vi "Mag calib routine.vi"(7 "Norm field":sgl format="%#_13g", 8 "Error In":errorcluster, 10 "Uncalibrated data":sgl[][](array[numeric])) -> (0 "Error Out":errorcluster, 1 "Calib data":T1, 2 "Calib data":sgl[](array[numeric]), 3 "Ainverse":sgl[][](array[numeric]))   [LabVIEW 2016]
uses:
  Typedef/Mag bit depth.ctl
  <vilib>/Analysis/Matrix/Datatypes/RealMatrix.ctl
  <vilib>/Analysis/baseanly.llb/Real A x B.vi
  <vilib>/Analysis/_algsub.llb/Real PseudoInverse Matrix.vi
  <vilib>/Analysis/7linalg.llb/Real Matrix Square Root.vi
  <vilib>/Analysis/7linalg.llb/Real Transpose Matrix.vi
  <vilib>/Analysis/Matrix/Numeric/Conversions/Array To Matrix - RA2.vi
  <vilib>/Analysis/Matrix/Numeric/Subtract/Subtract - RM,RM.vi
  <vilib>/Analysis/baseanly.llb/Real Inverse Matrix.vi
  <vilib>/Analysis/7linalg.llb/Real Eigenvalues and Vectors.vi
  <vilib>/Analysis/Matrix/Numeric/Absolute Value/Absolute Value - CM.vi
  <vilib>/Analysis/Matrix/Numeric/Subtract/Subtract (Elementwise) - RM,R.vi
  <vilib>/Analysis/Matrix/Numeric/Square Root/Square Root - RM.vi
  <vilib>/Analysis/Matrix/Numeric/Conversions/Matrix To Array - RM.vi
  <vilib>/Analysis/Matrix/Numeric/Multiply/Multiply - CM,C.vi
  <vilib>/Analysis/Matrix/Numeric/Conversions/Matrix To Array - CM.vi
  <vilib>/Analysis/Matrix/NI_Matrix.lvlib
  <vilib>/Analysis/NI_AALBase.lvlib
  <vilib>/Analysis/NI_AALPro.lvlib
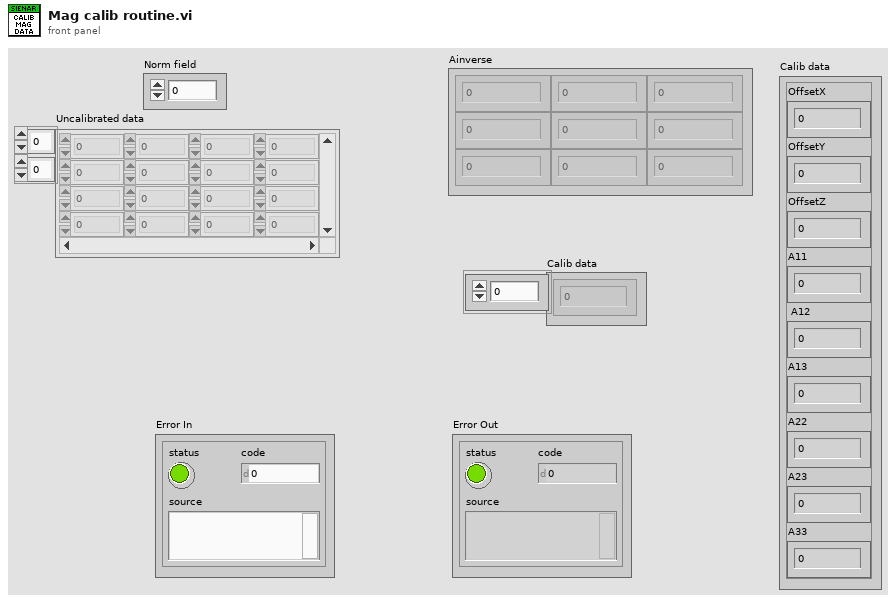
[diagram p1: front panel]
types:
  T1 = cluster{"OffsetX":i16, "OffsetY":i16, "OffsetZ":i16, "A11":sgl, " A12":sgl, "A13":sgl, "A22":sgl, "A23":sgl, "A33":sgl}
  T2 = typedef "Mag bit depth.ctl" = enum16{"14bit", "16bit"}
  T3 = typedef "NI_Matrix.lvlib/RealMatrix.ctl" = dbl[][]
  T4 = typedef "NI_Matrix.lvlib/ComplexMatrix.ctl" = cdb[][]
  T5 = cluster{i16, i16, i16, "Complex Matrix Element":sgl, "Complex Matrix Element":sgl, "Complex Matrix Element":sgl, "Complex Matrix Element":sgl, "Complex Matrix Element":sgl, "Complex Matrix Element":sgl}
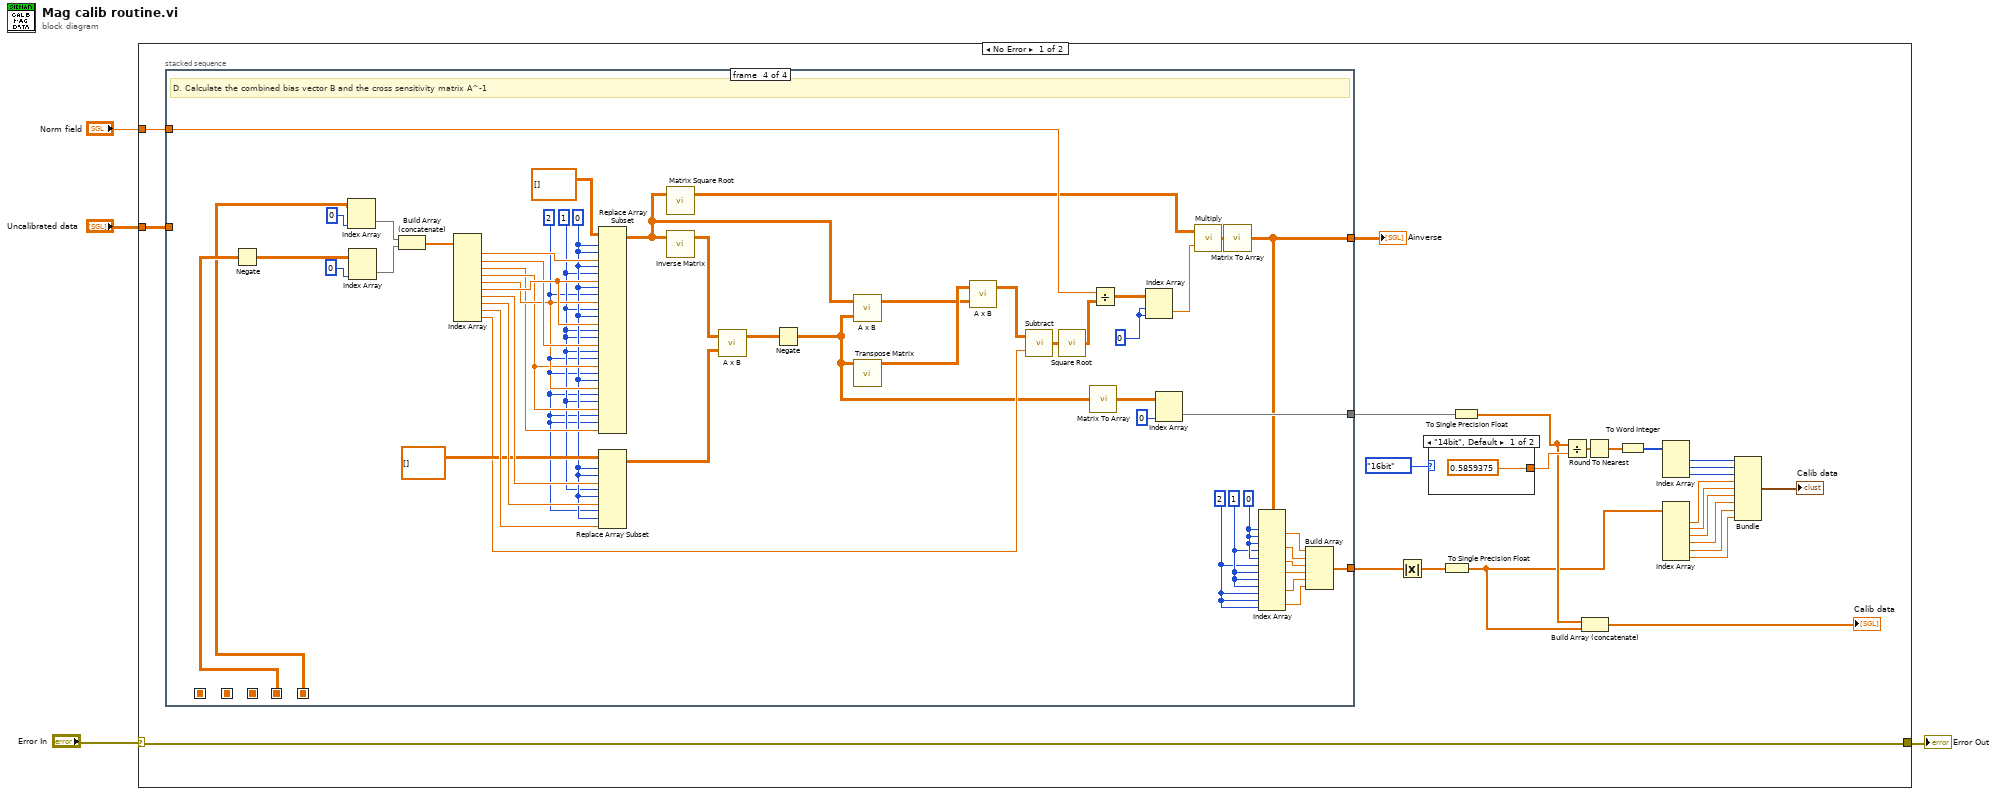
[diagram p0: block diagram]
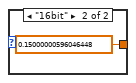
[diagram p2: hidden frame]
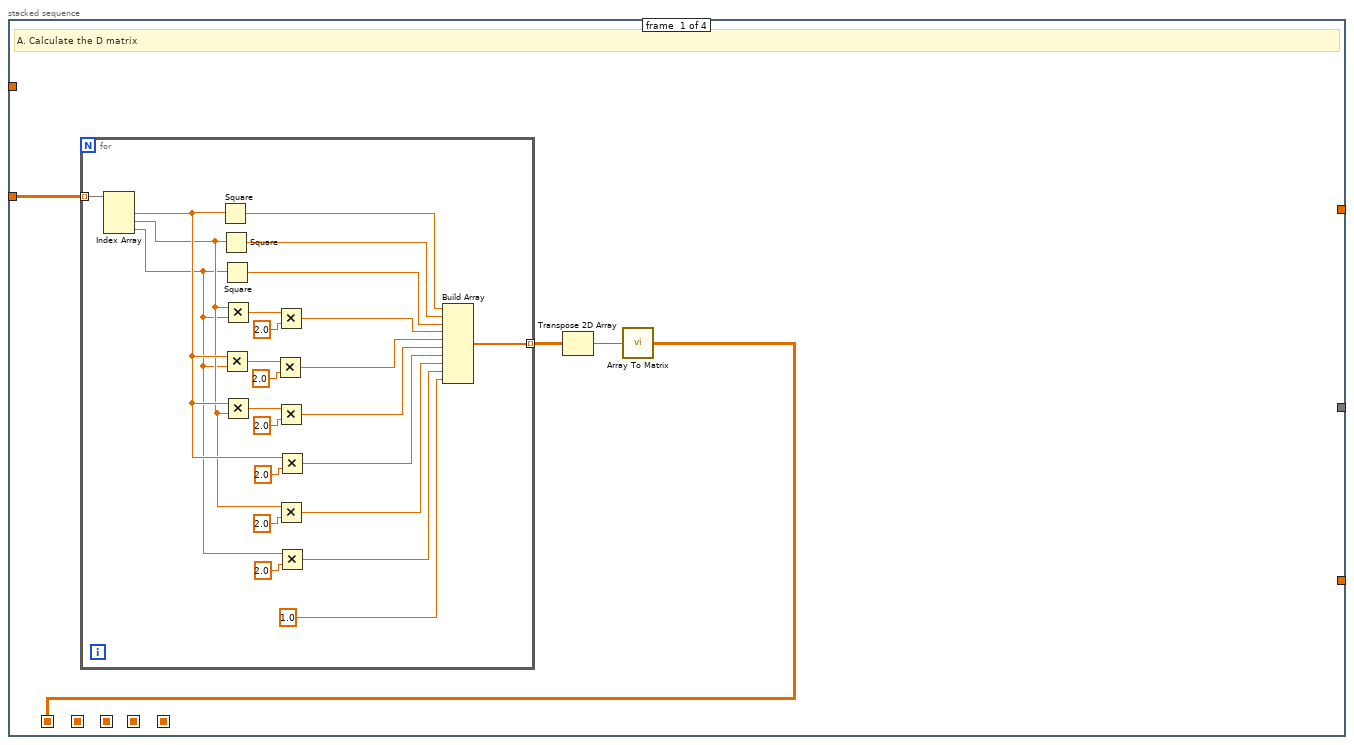
[diagram p3: hidden frame]
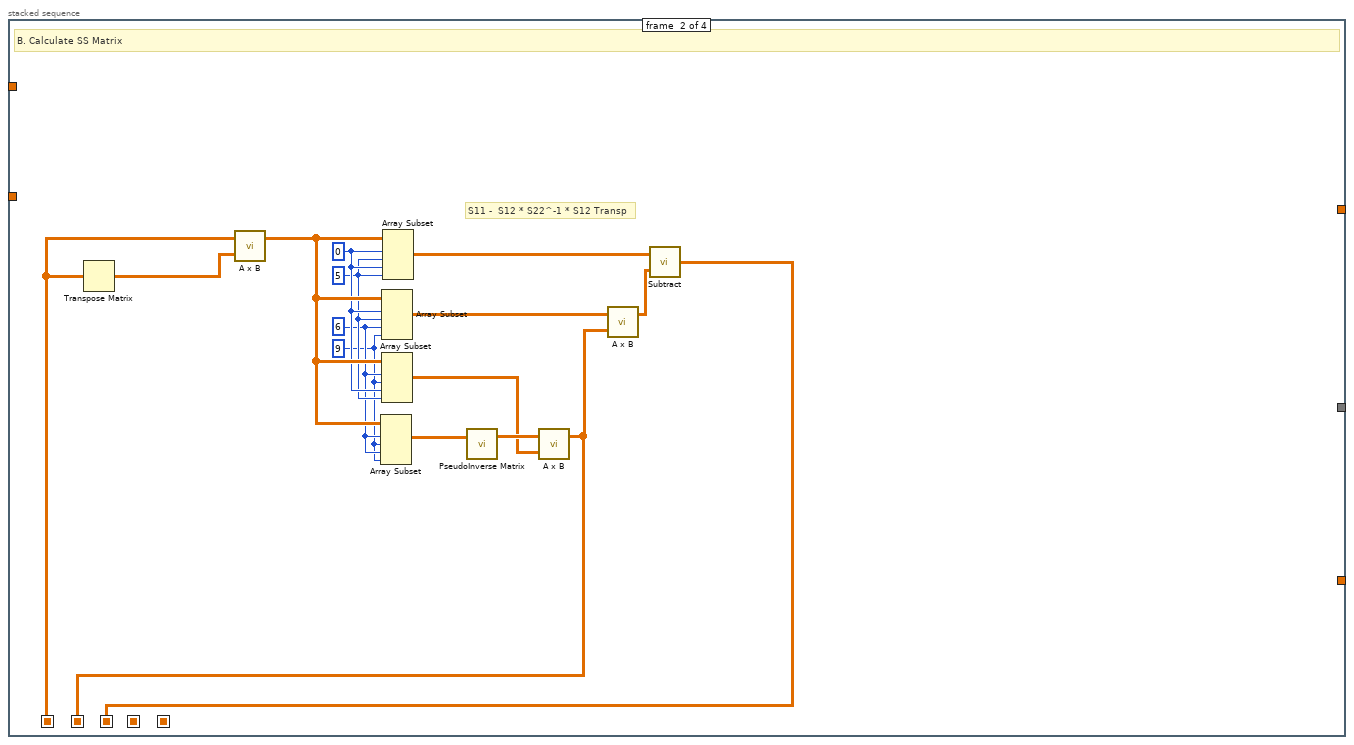
[diagram p4: hidden frame]
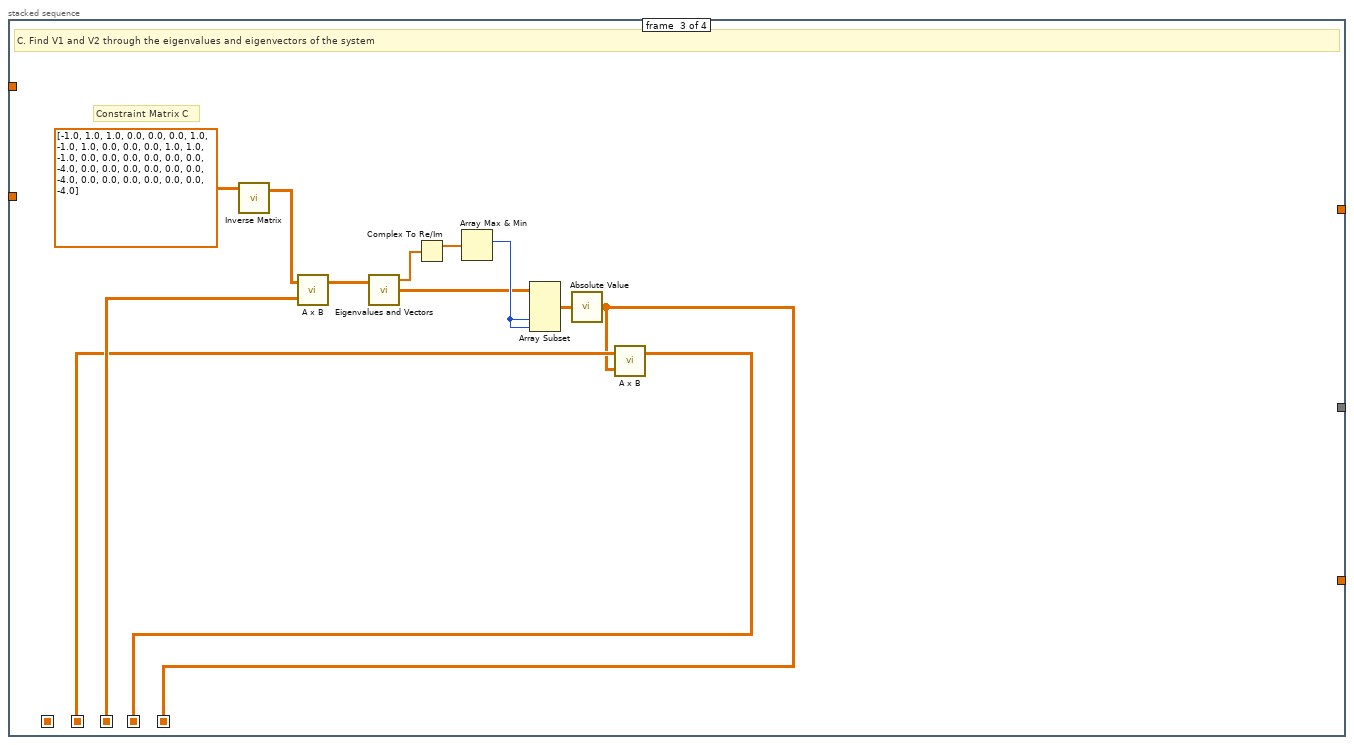
[diagram p5: hidden frame]
diagram:
  n1 = case shown="No Error" "Error In" {
    selector: "Error In" -> [w26 w140]
    tunnel: "Norm field" -> [w29 _]
    tunnel: "Uncalibrated data" -> [w27 _]
    tunnel: [w26 w140] -> w1
    frame No Error {
      n2 = stacked-sequence {
        seq-local: [w33 _ _ _] -> [_ w68 _ _]
        seq-local: [_ w61 _ _] -> [_ _ w85 _]
        seq-local: [_ w60 _ _] -> [_ _ w77 _]
        seq-local: [_ _ w76 _] -> [_ _ _ w139]
        seq-local: [_ _ w75 _] -> [_ _ _ w138]
        tunnel: w27 -> [w32 _ _ _]
        tunnel: w29 -> [_ _ _ w110]
        tunnel: [_ _ _ w97] -> w28
        tunnel: [_ _ _ w99] -> w21
        tunnel: [_ _ _ w87] -> w23
        frame #0 {
          # "A. Calculate the D matrix"
          n3 = for {
            tunnel: w32 -> [w59] mode=indexing
            tunnel: [w36] -> w35 mode=indexing
            n4 = Index Array(array=w59) -> (element #1=w49:sgl, element #2=w48:sgl, element #3=w47:sgl)  [unwired: 3 in]
            n5 = Square(x=w49) -> (x^2=w46:sgl)
            n6 = Square(x=w48) -> (x^2=w45:sgl)
            n7 = Square(x=w47) -> (x^2=w44:sgl)
            n8 = Multiply(x=w49, y=w47) -> (x*y=w56:sgl)
            n9 = Multiply(x=w48, y=w47) -> (x*y=w58:sgl)
            n10 = Multiply(x=w49, y=w48) -> (x*y=w54:sgl)
            n11 = Multiply(x=w56, y=2.0) -> (x*y=w42:dbl)
            n12 = Multiply(x=w58, y=2.0) -> (x*y=w43:dbl)
            n13 = Multiply(x=w54, y=2.0) -> (x*y=w41:dbl)
            n14 = Multiply(x=w48, y=2.0) -> (x*y=w39:dbl)
            n15 = Multiply(x=w49, y=2.0) -> (x*y=w40:dbl)
            n16 = Multiply(x=w47, y=2.0) -> (x*y=w38:dbl)
            n17 = Build Array(w46, w45, w44, w43, w42, w41, w40, w39, w38, 1.0) -> (w36:dbl[])
          }
          n18 = Transpose 2D Array(2D array=w35) -> (transposed array=w34:dbl[][])
          n19 = call-poly <vilib>:"Array To Matrix.vi"("Real 2D Array"=w34) -> ("Real Matrix"=w33:T3)
        }
        frame #1 {
          w69 = 9 ("column N")
          w70 = 6 ("column 1")
          w72 = 0 ("row 1")
          w71 = 5 ("row N")
          # "S11 -  S12 * S22^-1 * S12 Transp"
          # "B. Calculate SS Matrix"
          n20 = Transpose Matrix(1:w68) -> (0:w74:T3)
          n21 = call-poly <vilib>:"A x B.vi"("B"=w74, "A"=w68) -> ("A x B"=w73:T3)  [unwired: 1 out]
          n22 = Array Subset(array=w73, index (row)=w70, length (row)=w69, index (col)=w70, length (col)=w69) -> (w67:T3)
          n23 = Array Subset(array=w73, index (row)=w72, length (row)=w71, index (col)=w70, length (col)=w69) -> (w65:T3)
          n24 = Array Subset(array=w73, index (row)=w70, length (row)=w69, index (col)=w72, length (col)=w71) -> (w63:T3)
          n25 = Array Subset(array=w73, index (row)=w72, length (row)=w71, index (col)=w72, length (col)=w71) -> (w66:T3)
          n26 = call-poly <vilib>:"PseudoInverse Matrix.vi"("Input Matrix"=w67) -> ("PseudoInverse Matrix"=w64:T3)  [unwired: 1 in, 1 out]
          n27 = call-poly <vilib>:"A x B.vi"("B"=w63, "A"=w64) -> ("A x B"=w60:T3)  [unwired: 1 out]
          n28 = call-poly <vilib>:"A x B.vi"("B"=w60, "A"=w65) -> ("A x B"=w62:T3)  [unwired: 1 out]
          n29 = call-poly <vilib>:"Subtract.vi"("Real Matrix B"=w62, "Real Matrix A"=w66) -> ("A - B"=w61:T3)
        }
        frame #2 {
          # "Constraint Matrix C"
          # "C. Find V1 and V2 through the eigenvalues and eigenvectors of the system"
          n30 = call-poly <vilib>:"Inverse Matrix.vi"("Input Matrix"=T3 [[-1.0, 1.0, 1.0, 0.0, 0.0, 0.0], [1.0, -1.0, 1.0, 0.0, 0.0, 0.0], [1.0, 1.0, -1.0, 0.0, 0.0, 0.0], [0.0, 0.0, 0.0, -4.0, 0.0, 0.0], [0.0, 0.0, 0.0, 0.0, -4.0, 0.0], [0.0, 0.0, 0.0, 0.0, 0.0, -4.0]] ("Real Matrix")) -> ("Inverse Matrix"=w84:T3)  [unwired: 1 in, 1 out]
          n31 = call-poly <vilib>:"A x B.vi"("B"=w85, "A"=w84) -> ("A x B"=w83:T3)  [unwired: 1 out]
          n32 = call-poly <vilib>:"Eigenvalues and Vectors.vi"("Input Matrix"=w83) -> ("Eigenvectors"=w79:T4, "Eigenvalues"=w82:cdb[])  [unwired: 2 in, 1 out]
          n33 = Complex To Re/Im(x + iy=w82) -> (x=w81:dbl[])  [unwired: 1 out]
          n34 = Array Max & Min(array=w81) -> (max index (indices)=w80:i32)  [unwired: 3 out]
          n35 = Array Subset(array=w79, index (col)=w80, length (col)=w80) -> (w78:T4)  [unwired: 2 in]
          n36 = call-poly <vilib>:"Absolute Value.vi"("Complex Matrix A"=w78) -> ("|A|"=w75:T3)
          n37 = call-poly <vilib>:"A x B.vi"("B"=w75, "A"=w77) -> ("A x B"=w76:T3)  [unwired: 1 out]
        }
        frame #3 {
          w94 = 2 ("index (col)")
          w95 = 1 ("index (col)")
          w96 = 0 ("index (row)")
          w108 = 0
          w118 = 2
          w119 = 1
          w120 = 0 ("disabled index (row)")
          # "D. Calculate the combined bias vector B and the cross sensitivity matrix A^-1"
          n38 = Negate(x=w139) -> (-x=w137:T3)
          n39 = Index Array(array=w138, index (col)=0 ("disabled index (col)")) -> (element=w134:dbl[])  [unwired: 1 in]
          n40 = Index Array(array=w137, index (col)=0 ("disabled index (col)")) -> (element=w133:dbl[])  [unwired: 1 in]
          n41 = Build Array (concatenate)(w134, w133) -> (w132:dbl[])
          n42 = Index Array(array=w132) -> (element #1=w130:dbl, element #2=w128:dbl, element #3=w125:dbl, element #4=w126:dbl, element #5=w127:dbl, element #6=w129:dbl, element #7=w124:dbl, element #8=w123:dbl, element #9=w122:dbl, element #10=w113:dbl)  [unwired: 10 in]
          n43 = Replace Array Subset(array=T3 [] ("matrix"), new element #1=w130, index (row) #1=w120, index (col) #1=w120, new element #2=w129, index (row) #2=w120, index (col) #2=w119, new element #3=w127, index (row) #3=w120, index (col) #3=w118, new element #4=w129, index (row) #4=w119, index (col) #4=w120, new element #5=w128, index (row) #5=w119, index (col) #5=w119, new element #6=w126, index (row) #6=w119, index (col) #6=w118, new element #7=w127, index (row) #7=w118, index (col) #7=w120, new element #8=w126, index (row) #8=w118, index (col) #8=w119, new element #9=w125, index (row) #9=w118, index (col) #9=w118) -> (w104:T3)
          n44 = Replace Array Subset(array=T3 [] ("matrix"), new element #1=w124, index (row) #1=w120, index (col) #1=w120, new element #2=w123, index (row) #2=w119, index (col) #2=w120, new element #3=w122, index (row) #3=w118, index (col) #3=w120) -> (w117:T3)
          n45 = call-poly <vilib>:"Matrix Square Root.vi"("Input Matrix"=w104) -> ("Matrix Square Root"=w106:T4)  [unwired: 1 in, 1 out]
          n46 = call-poly <vilib>:"Inverse Matrix.vi"("Input Matrix"=w104) -> ("Inverse Matrix"=w103:T3)  [unwired: 1 in, 1 out]
          n47 = call-poly <vilib>:"A x B.vi"("B"=w117, "A"=w103) -> ("A x B"=w105:T3)  [unwired: 1 out]
          n48 = Negate(x=w105) -> (-x=w101:T3)
          n49 = call-poly <vilib>:"A x B.vi"("B"=w101, "A"=w104) -> ("A x B"=w115:T3)  [unwired: 1 out]
          n50 = call-poly <vilib>:"Transpose Matrix.vi"("Input Matrix"=w101) -> ("Matrix Transpose"=w116:T3)  [unwired: 9 in, 1 out]
          n51 = call-poly <vilib>:"A x B.vi"("B"=w115, "A"=w116) -> ("A x B"=w114:T3)  [unwired: 1 out]
          n52 = call-poly <vilib>:"Subtract.vi"("Real Scalar c"=w113, "Real Matrix A"=w114) -> ("A - c"=w112:T3)
          n53 = call-poly <vilib>:"Square Root.vi"("Real Matrix A"=w112) -> ("sqrt(A)"=w111:T4)
          n54 = call-poly <vilib>:"Matrix To Array.vi"("Real Matrix"=w101) -> ("Real 2D Array"=w100:dbl[][])
          n55 = Divide(x=w110, y=w111) -> (x/y=w109:T4)
          n56 = Index Array(array=w109, index (row)=w108, index (col)=w108) -> (element=w107:cdb)
          n57 = Index Array(array=w100, index (col)=0 ("disabled index (col)")) -> (element=w99:dbl[])  [unwired: 1 in]
          n58 = call-poly <vilib>:"Multiply.vi"("Complex Scalar c"=w107, "Complex Matrix A"=w106) -> ("A * c"=w102:T4)
          n59 = call-poly <vilib>:"Matrix To Array.vi"("Complex Matrix"=w102) -> ("Complex 2D Array"=w97:cdb[][])
          n60 = Index Array(array=w97, index (row) #1=w96, index (col) #1=w96, index (row) #2=w96, index (col) #2=w95, index (row) #3=w96, index (col) #3=w94, index (row) #4=w95, index (col) #4=w95, index (row) #5=w95, index (col) #5=w94, index (row) #6=w94, index (col) #6=w94) -> (element #1=w93:cdb, element #2=w92:cdb, element #3=w91:cdb, element #4=w90:cdb, element #5=w89:cdb, element #6=w88:cdb)
          n61 = Build Array(w93, w92, w91, w90, w89, w88) -> (w87:cdb[])
        }
      }
      "Ainverse" <- w28
      n62 = Absolute Value(x=w23) -> (abs(x)=w22:dbl[])
      n63 = case shown="\"14bit\", Default" Mag_bit_depth."16bit" ("Mag bit depth") {
        tunnel: [sgl 0.5859375 sgl 0.15] -> w24
        frame "14bit", Default {
        }
        frame "16bit" {
        }
      }
      n64 = To Single Precision Float(number=w22) -> (single precision float=w11:sgl[])
      n65 = To Single Precision Float(number=w21) -> (single precision float=w20:sgl[])
      n66 = Divide(x=w20, y=w24) -> (x/y=w18:sgl[])
      n67 = Build Array (concatenate)(w20, w11) -> (→"Calib data":sgl[])
      n68 = Round To Nearest(number=w18) -> (nearest integer value=w16:sgl[])
      n69 = To Word Integer(number=w16) -> (16bit integer=w15:i16[])
      n70 = Index Array(array=w15) -> (element #1=w14:i16, element #2=w13:i16, element #3=w12:i16)  [unwired: 3 in]
      n71 = Index Array(array=w11) -> (element #1=w10:sgl, element #2=w9:sgl, element #3=w8:sgl, element #4=w7:sgl, element #5=w6:sgl, element #6=w5:sgl)  [unwired: 6 in]
      n72 = Bundle(w14, w13, w12, "Complex Matrix Element"=w10, "Complex Matrix Element"=w9, "Complex Matrix Element"=w8, "Complex Matrix Element"=w7, "Complex Matrix Element"=w6, "Complex Matrix Element"=w5) -> (→"Calib data":T5)  [unwired: 1 in]
    }
    frame Error {
    }
  }
  "Error Out" <- w1
